vi "Smoothed Frame Rate.vi"(5 "Feedback In":T1, 6 "Alpha":dbl=0.1) -> (1 "Feedback Out":T1, 2 "Frame Rate":dbl)   [LabVIEW 2010]
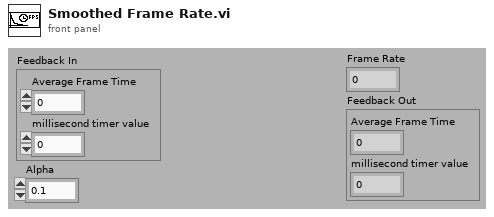
[diagram p1: front panel]
types:
  T1 = cluster{"Average Frame Time":dbl, "millisecond timer value":u32}
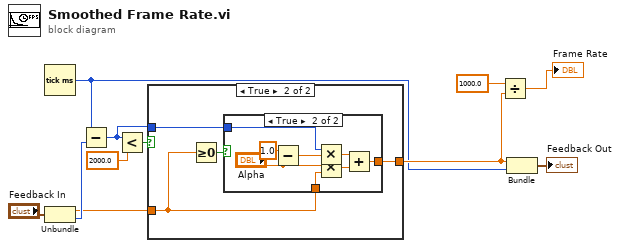
[diagram p0: block diagram]
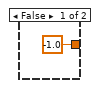
[diagram p2: hidden frame]
diagram:
  n1 = Tick Count (ms)() -> (millisecond timer value=w2:u32)
  n2 = Unbundle("Feedback In") -> ("Average Frame Time"=w1:dbl, "millisecond timer value"=w4:u32)
  n3 = Subtract(x=w2, y=w4) -> (x-y=w3:u32)
  n4 = Less?(x=w3, y=2000.0) -> (x < y?=w8:bool)
  n5 = case shown="True" w8 {
    tunnel: [-1.0 w16] -> w7
    tunnel: w3 -> [_ w15]
    tunnel: w1 -> [_ w14]
    frame False {
    }
    frame True {
      n6 = Greater Or Equal To 0?(x=w14) -> (x >= 0?=w13:bool)
      n7 = case shown="True" w13 {
        tunnel: [w17 w20] -> w16
        tunnel: w15 -> [w17 w19]
        tunnel: w14 -> [_ w18]
        frame False {
        }
        frame True {
          n8 = Subtract(x=1.0, y="Alpha") -> (x-y=w22:dbl)
          n9 = Multiply(x=w19, y="Alpha") -> (x*y=w25:dbl)
          n10 = Multiply(x=w22, y=w18) -> (x*y=w24:dbl)
          n11 = Add(x=w25, y=w24) -> (x+y=w20:dbl)
        }
      }
    }
  }
  n12 = Divide(x=1000.0, y=w7) -> (x/y=→"Frame Rate":dbl)
  n13 = Bundle(w7, "millisecond timer value"=w2) -> (→"Feedback Out":cluster{dbl, "millisecond timer value":u32})  [unwired: 1 out]
